vi "Read current unit ID.vi"(8 "error in (no error)":errorcluster, 11 "serial data unit in":refnum<class "Serial Data Unit.lvclass">) -> (0 "error out":errorcluster, 2 "request unit ID":u8, 3 "serial data unit out":refnum<class "Serial Data Unit.lvclass">)   [LabVIEW 2020, in "SubVIs.lvlib" / "Serial Data Unit.lvclass"]
uses:
  <vilib>/Modbus/subvis/Transmission Data Unit (ADU)/Serial Data Unit/Serial Data Unit.lvclass
  <vilib>/Modbus/subvis/Transmission Data Unit (ADU)/Serial Data Unit/Serial Data Unit.lvclass/Serial Data Unit.ctl
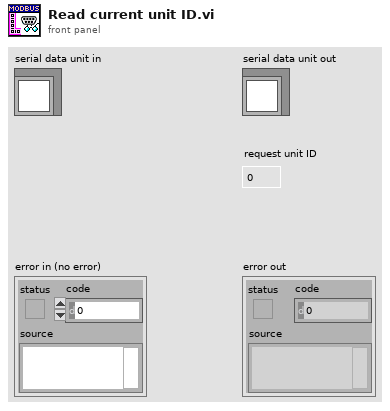
[diagram p1: front panel]
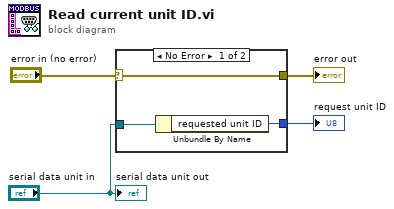
[diagram p0: block diagram]
diagram:
  n1 = case shown="No Error" "error in (no error)" {
    selector: "error in (no error)" -> [w5 w8]
    tunnel: "serial data unit in" -> [w7 _]
    tunnel: [w6 _] -> w3
    tunnel: [w5 w8] -> w1
    frame No Error {
      n2 = Unbundle By Name(w7) -> ("requested unit ID"=w6:u8)
    }
    frame Error {
    }
  }
  "error out" <- w1
  "request unit ID" <- w3
  "serial data unit out" <- "serial data unit in"
